vi "GFITS_ReplicateRemoteDir.vi"(7 "error in":errorcluster, 8 "replicate remote dir?":bool, 9 "alternative local dir":path, 10 "remote dir":path) -> (0 "error":errorcluster, 3 "local dir  out":path)   [LabVIEW 2016]
doc: "This VI will examine the directory given and will create it if it does not exists."
panel:
  in  "sep":string="/"
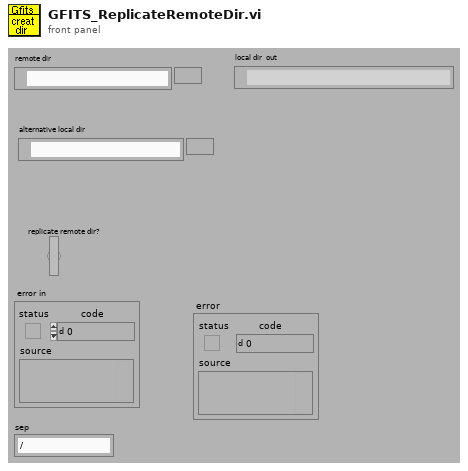
[diagram p1: front panel]
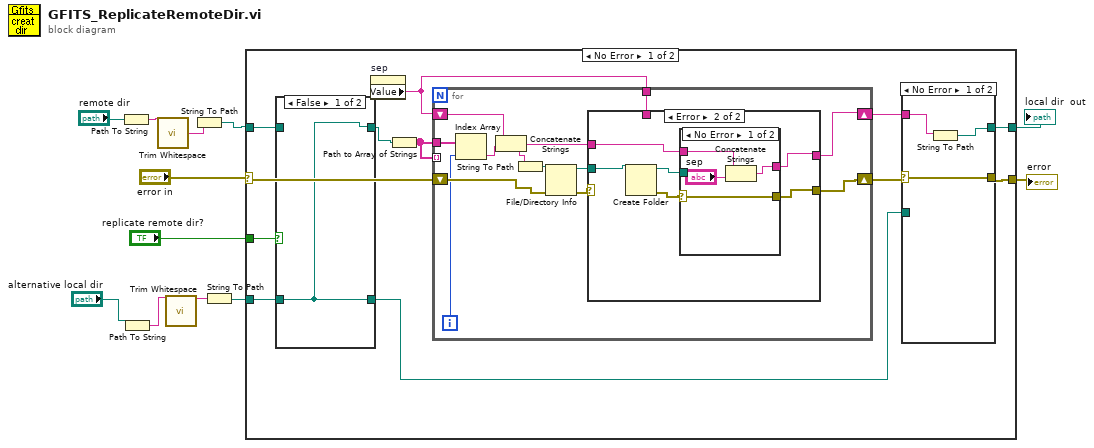
[diagram p0: block diagram]
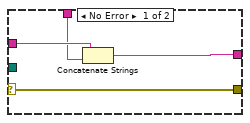
[diagram p4: hidden frame]
diagram:
  n1 = Path To String(path="remote dir") -> (string=w3:string)
  n2 = Path To String(path="alternative local dir") -> (string=w7:string)
  n3 = call <vilib>:"Trim Whitespace.vi"("string"=w3) -> ("trimmed string"=w2:string)  [unwired: 1 in]
  n4 = call <vilib>:"Trim Whitespace.vi"("string"=w7) -> ("trimmed string"=w6:string)  [unwired: 1 in]
  n5 = String To Path(string=w2) -> (path=w1:path)
  n6 = String To Path(string=w6) -> (path=w5:path)
  n7 = case shown="No Error" "error in" {
    selector: "error in" -> [w18 w61]
    tunnel: [w23 w62] -> w12
    tunnel: w1 -> [w17 _]
    tunnel: w5 -> [w15 w62]
    tunnel: [w22 w61] -> w11
    tunnel: "replicate remote dir?" -> [w19 _]
    frame No Error {
      n8 = case shown="False" w19 {
        tunnel: w17 -> [_ w27]
        tunnel: [w25 w27] -> w16
        tunnel: w15 -> [w25 w26]
        tunnel: [w25 w26] -> w14
        frame False {
        }
        frame True {
        }
      }
      n9 = property on="sep" class="Str"() -> ("Value"=w13:string)  [unwired: 2 in, 2 out]
      n10 = Path to Array of Strings(0:w16) -> (2:w21:string[])  [unwired: 1 out]
      n11 = for {
        shift-right: [w40] -> w24
        shift-left: w18 -> [w41]
        shift-right: [w35] -> w20
        shift-left: w13 -> [w36]
        tunnel: w21 -> [w34]
        tunnel: w21 -> [_] mode=indexing
        tunnel: w13 -> [w33]
        i -> [w39]
        n12 = Index Array(array=w34, index=w39) -> (element=w37:string)
        n13 = Concatenate Strings(w36, w37) -> (w38:string)
        n14 = String To Path(string=w38) -> (path=w44:path)
        n15 = File/Directory Info(path=w44, error in=w41) -> (path out=w42:path, error out=w43:errorcluster)  [unwired: 5 out]
        n16 = case shown="Error" w43 {
          selector: w43 -> [w48 _]
          tunnel: [w46 w52] -> w35
          tunnel: w42 -> [_ w54]
          tunnel: [w48 w51] -> w40
          tunnel: w38 -> [w47 w50]
          tunnel: w33 -> [w45 _]
          frame No Error {
            n17 = Concatenate Strings(w47, w45) -> (w46:string)
          }
          frame Error {
            n18 = Create Folder(path (use dialog)=w54) -> (created path=w49:path, error out=w53:errorcluster)  [unwired: 1 in, 2 out]
            n19 = case shown="No Error" w53 {
              selector: w53 -> [w58 w60]
              tunnel: [w56 w59] -> w52
              tunnel: [w58 w60] -> w51
              tunnel: w50 -> [w57 w59]
              tunnel: w49 -> [_ _]
              frame No Error {
                n20 = Concatenate Strings(w57, "sep") -> (w56:string)
              }
              frame Error {
              }
            }
          }
        }
      }
      n21 = case shown="No Error" w24 {
        selector: w24 -> [w30 w31]
        tunnel: [w28 w32] -> w23
        tunnel: w14 -> [_ w32]
        tunnel: [w30 w31] -> w22
        tunnel: w20 -> [w29 _]
        frame No Error {
          n22 = String To Path(string=w29) -> (path=w28:path)
        }
        frame Error {
        }
      }
    }
    frame Error {
    }
  }
  "local dir  out" <- w12
  "error" <- w11
